vi "FTP_UploadFile.vi"(1 "error in":errorcluster, 3 "Passive Port":T1, 4 "file path":path) -> (0 "error out":errorcluster)   [LabVIEW 2012]
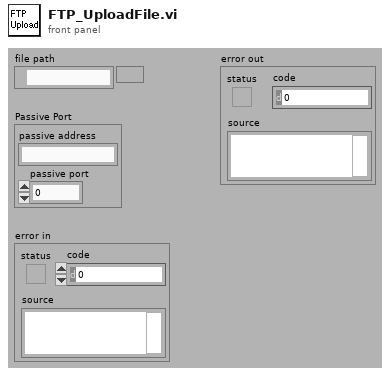
[diagram p1: front panel]
types:
  T1 = cluster{"passive address":string, "passive port":u16}
  T2 = enum16{"open", "replace", "create", "open or create", "replace or create", "replace or create with confirmation"}
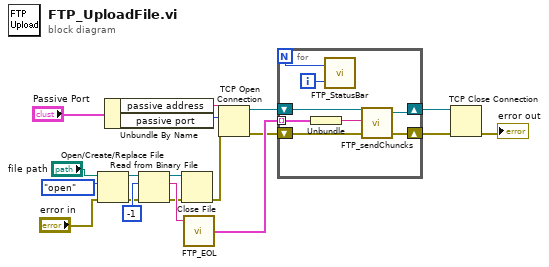
[diagram p0: block diagram]
diagram:
  n1 = Open/Create/Replace File(file path (use dialog)="file path", error in="error in", operation (0:open)=T2."open") -> (refnum out=w5:refnum<file>, error out=w4:errorcluster)  [unwired: 4 out]
  n2 = Unbundle By Name("Passive Port") -> ("passive address"=w2:string, "passive port"=w3:u16)
  n3 = Read from Binary File(8:w4, 10:-1 ("count (1)"), 11:w5) -> (0:w6:errorcluster, 2:w11:string, 3:w7:refnum<file>)  [unwired: 4 out]
  n4 = Close File(refnum=w7, error in=w6) -> (error out=w12:errorcluster)  [unwired: 1 out]
  n5 = call <userlib>:"FTP_EOL.vi"("String"=w11) -> ("chuncks"=w17:cluster{"result string":string}[])  [unwired: 1 in, 1 out]
  n6 = TCP Open Connection(address=w2, remote port or service name=w3, error in (no error)=w12) -> (connection ID=w13:refnum<k5>, error out=w14:errorcluster)  [unwired: 2 out]
  n7 = for {
    N -> [w20]
    tunnel: w17 -> [w23] mode=indexing
    shift-right: [w24] -> w16
    shift-left: w13 -> [w27]
    shift-right: [w25] -> w15
    shift-left: w14 -> [w26]
    i -> [w21]
    n8 = Unbundle(w23) -> ("result string"=w22:string)
    n9 = call <userlib>:"FTP_StatusBar.vi"("i"=w21, "N"=w20) -> ()  [unwired: 1 in, 1 out]
    n10 = call <userlib>:"FTP_sendChuncks.vi"("error in (no error)"=w26, "data in"=w22, "connection ID"=w27) -> ("error out"=w25:errorcluster, "connection ID out"=w24:refnum<k5>)  [unwired: 1 out]
  }
  n11 = TCP Close Connection(connection ID=w16, error in (no error)=w15) -> (error out=→"error out":errorcluster)  [unwired: 2 out]
